vi "MH_DataProcThread.vi"(10 "MH_VisThread_QRef":T1, 11 "MH_DataProcThread_QRef":T2) -> ()   [LabVIEW 2017]
uses:
  Types/MH_DataProcThread_QRef.ctl
  Types/MH_DataProcThread_QData.ctl
  Types/MH_DataProcThread_QCmds.ctl
  Types/MH_VisThread_QRef.ctl
  Types/MH_VisThread_QData.ctl
  Types/MH_VisThread_QCmds.ctl
  Types/MH_DataProcThread_Data.ctl
  MH_InsertIntoTimeTrace.vi
  MH_CalcTimeTrace.vi
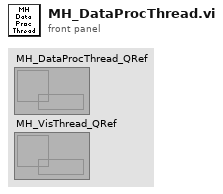
[diagram p1: front panel]
types:
  T1 = typedef "MH_VisThread_QRef.ctl" = refnum<queue>
  T2 = typedef "MH_DataProcThread_QRef.ctl" = refnum<queue>
  T3 = typedef "MH_DataProcThread_Data.ctl" = cluster{"TimeTraces":u32[][], "BitShift":i16, "NumChannels":i32, "Total bin":u64, "Bin":i32, "HistAcqTime":i32, "HistoTime":u64, "Histos":u32[][], "HistosZero":u32[][], "ChannelsZero":u32[]}
  T4 = typedef "MH_VisThread_QCmds.ctl" = enum16{"_none_", "Resol", "nChannels", "DeltaT", "Histo", "TTrace", "Status"}
  T5 = typedef "MH_DataProcThread_QData.ctl" = cluster{"Cmd":T6, "nActual":i32, "Buffer":u32[], "TickCount":u32, "Param":i32}
  T6 = typedef "MH_DataProcThread_QCmds.ctl" = enum16{"Exit", "Proc", "Init", "SetShift", "SetNumChannels", "SetHistAcqTime"}
  T7 = typedef "MH_VisThread_QData.ctl" = cluster{"Histos":u32[][], "Cmd":T4, "TimeTrace":u32[][], "Bin":i32, "Total bin":u64, "Status":string, "Resol":dbl, "DeltaT":dbl, "nChannels":i32}
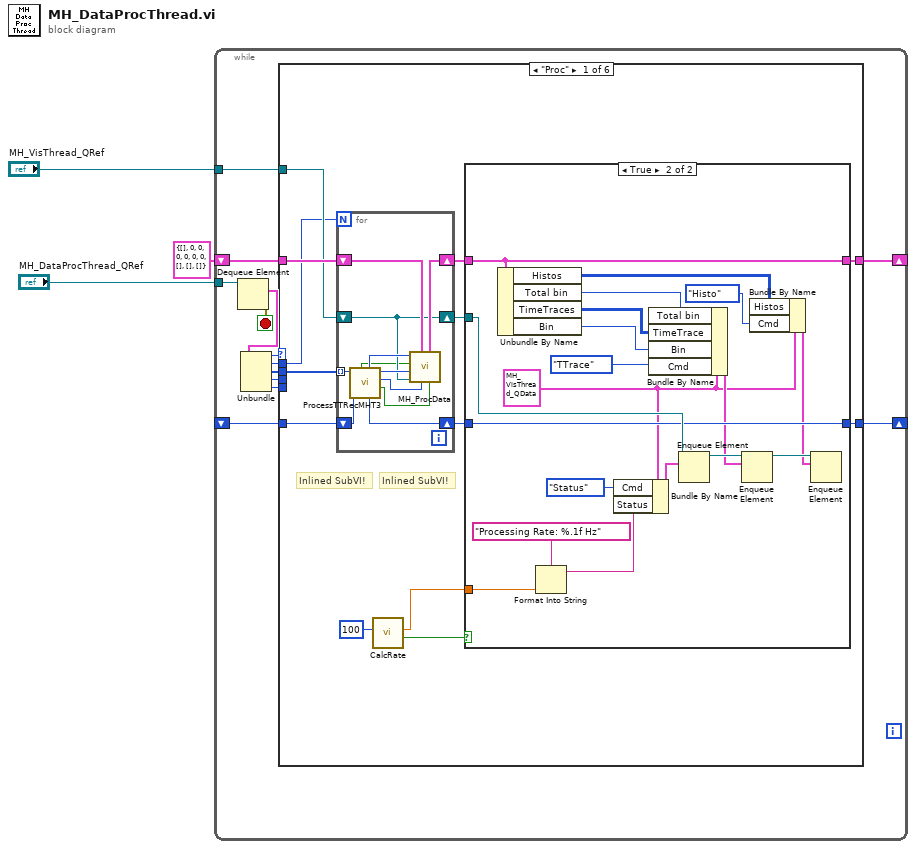
[diagram p0: block diagram]
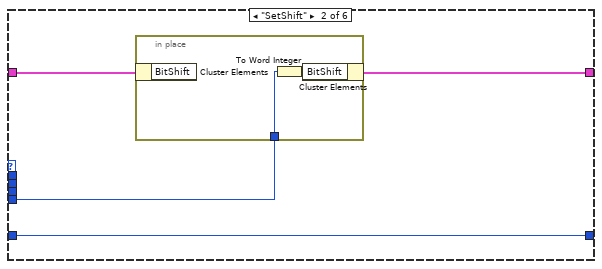
[diagram p3: hidden frame]
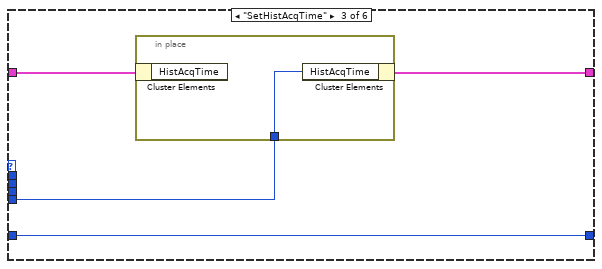
[diagram p4: hidden frame]
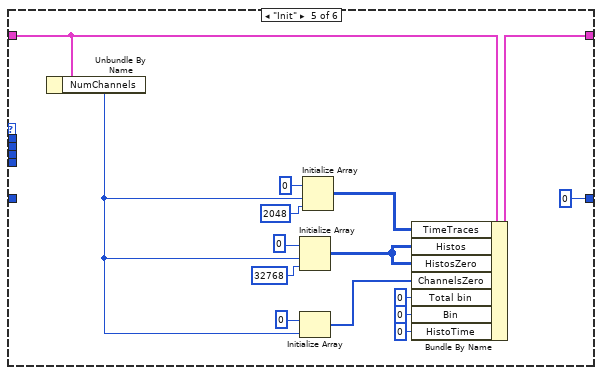
[diagram p6: hidden frame]
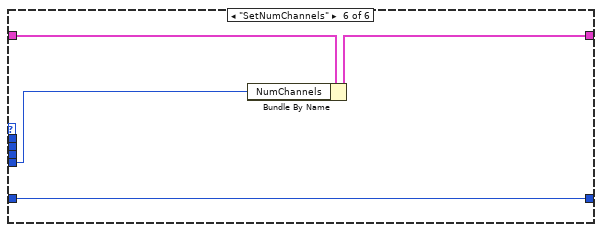
[diagram p7: hidden frame]
diagram:
  n1 = while {
    tunnel: "MH_DataProcThread_QRef" -> [w5]
    shift-right: [w12] -> _
    shift-left: _ -> [w11]
    shift-right: [w10] -> _
    shift-left: T3 {"TimeTraces"=[], "BitShift"=0, "NumChannels"=0, "Total bin"=0, "Bin"=0, "HistAcqTime"=0, "HistoTime"=0, "Histos"=[], "HistosZero"=[], "ChannelsZero"=[]} ("RTData_out") -> [w9]
    tunnel: "MH_VisThread_QRef" -> [w4]
    stop <- w8 stop-if-true
    n2 = Dequeue Element(queue=w5) -> (element=w16:T5, error out=w8:errorcluster)  [unwired: 2 in, 2 out]
    n3 = Unbundle(w16) -> ("Cmd"=w15:T6, "nActual"=w14:i32, "Buffer"=w13:u32[], "TickCount"=w7:u32, "Param"=w6:i32)
    n4 = case shown="\"Proc\"" w15 {
      tunnel: w14 -> [w18 _ _ _ _ _]
      tunnel: w13 -> [w28 _ _ _ _ _]
      tunnel: [w20 w65 w71 w73 u64 0 ("ofl out") w90] -> w12
      tunnel: w11 -> [w29 w65 w71 w73 _ w90]
      tunnel: [w21 w63 w69 w74 w84 w92] -> w10
      tunnel: w9 -> [w25 w64 w70 w74 w83 w93]
      tunnel: w7 -> [_ _ _ _ _ _]
      tunnel: w6 -> [_ w62 w68 _ _ w91]
      tunnel: w4 -> [w24 _ _ _ _ _]
      frame "Proc" {
        # "Inlined SubVI!"
        # "Inlined SubVI!"
        n5 = for {
          N: w18 -> [_]
          tunnel: w28 -> [w59] mode=indexing
          shift-right: [w61] -> w19
          shift-left: w29 -> [w60]
          shift-right: [w58] -> w27
          shift-left: w25 -> [w55]
          shift-right: [w54] -> w26
          shift-left: w24 -> [w54]
          n6 = call "ProcessTTRecMHT3.vi"("oflcorr_in"=w60, "rawbits"=w59) -> ("is_marker"=w53:bool, "channel"=w51:u32, "dtime"=w56:u32, "oflcorr_out"=w61:u64, "truetime"=w57:u64, "is_photon"=w52:bool)  [unwired: 3 in, 1 out]
          n7 = call "MH_ProcData.vi"("isMarker"=w53, "Channel"=w51, "MHData in"=w55, "MH_VisThread_QRef"=w54, "dtime"=w56, "photon"=w52, "truetime"=w57) -> ("MHData out"=w58:T3)  [unwired: 4 in]
        }
        n8 = call "CalcRate.vi"("Refresh(ms)"=u32 100) -> ("updated?"=w23:bool, "Rate / Hz"=w17:dbl)  [unwired: 8 in, 1 out]
        n9 = case shown="True" w23 {
          tunnel: w27 -> [w31 w46]
          tunnel: w26 -> [_ w49]
          tunnel: [w31 w46] -> w21
          tunnel: [w30 w47] -> w20
          tunnel: w19 -> [w30 w47]
          tunnel: w17 -> [_ w32]
          frame False {
          }
          frame True {
            w36 = T7 {"Histos"=[], "Cmd"=enum."_none_", "TimeTrace"=[], "Bin"=0, "Total bin"=0, "Status"="", "Resol"=0.0, "DeltaT"=0.0, "nChannels"=0} ("element")
            n10 = Unbundle By Name(w46) -> ("Histos"=w35:u32[][], "Total bin"=w40:u64, "TimeTraces"=w39:u32[][], "Bin"=w38:i32)
            n11 = Format Into String(format string="Processing Rate: %.1f Hz", w32) -> (resulting string=w45:string)  [unwired: 2 in, 1 out]
            n12 = Bundle By Name(cluster=w36, "Cmd"=MH_VisThread_QCmds."Status", "Status"=w45) -> (w44:T7)
            n13 = Bundle By Name(cluster=w36, "Total bin"=w40, "TimeTrace"=w39, "Bin"=w38, "Cmd"=MH_VisThread_QCmds."TTrace") -> (w41:T7)
            n14 = Enqueue Element(queue=w49, element=w44) -> (queue out=w48:T1)  [unwired: 2 in, 2 out]
            n15 = Enqueue Element(queue=w48, element=w41) -> (queue out=w37:T1)  [unwired: 2 in, 2 out]
            n16 = Bundle By Name(cluster=w36, "Histos"=w35, "Cmd"=MH_VisThread_QCmds."Histo") -> (w33:T7)
            n17 = Enqueue Element(queue=w37, element=w33) -> ()  [unwired: 2 in, 3 out]
          }
        }
      }
      frame "SetShift" {
        n18 = in-place {
          in-place-border: w62 -> [w67]
          n19 = in-place-cluster #1(w64) -> ()  [unwired: 1 out]
          n20 = To Word Integer(number=w67) -> (16bit integer=w66:i16)
          n21 = in-place-cluster #1("BitShift"=w66) -> (w63:T3)
        }
      }
      frame "SetHistAcqTime" {
        n22 = in-place {
          in-place-border: w68 -> [w72]
          n23 = in-place-cluster #2(w70) -> ()  [unwired: 1 out]
          n24 = in-place-cluster #2("HistAcqTime"=w72) -> (w69:T3)
        }
      }
      frame "Exit", Default {
      }
      frame "Init" {
        n25 = Unbundle By Name(w83) -> ("NumChannels"=w75:i32)
        n26 = Initialize Array(u32 0, w75, 32768 ("dimension size")) -> (w79:u32[][])
        n27 = Initialize Array(u32 0, w75) -> (w77:u32[])
        n28 = Initialize Array(u32 0, w75, 2048 ("dimension size")) -> (w87:u32[][])
        n29 = Bundle By Name(cluster=w83, "TimeTraces"=w87, "Histos"=w79, "HistosZero"=w79, "ChannelsZero"=w77, "Total bin"=u64 0 ("Last total bin"), "Bin"=0 ("Last bin"), "HistoTime"=u64 0) -> (w84:T3)
      }
      frame "SetNumChannels" {
        n30 = Bundle By Name(cluster=w93, "NumChannels"=w91) -> (w92:T3)
      }
    }
  }
